vi "read_matrix_reshape.vi"   [LabVIEW 2012]
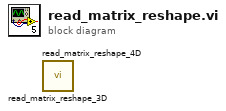
[diagram p0: block diagram]
diagram:
  n1 = call "read_matrix_reshape_4D.vi"() -> ()  [unwired: 11 in, 1 out]
  n2 = call "read_matrix_reshape_3D.vi"() -> ()  [unwired: 11 in, 1 out]
